vi "Open.vi"(8 "error in (no error)":errorcluster) -> (0 "error out":errorcluster, 3 "return type":i16)   [LabVIEW 2023]
uses:
  ps2000.dll
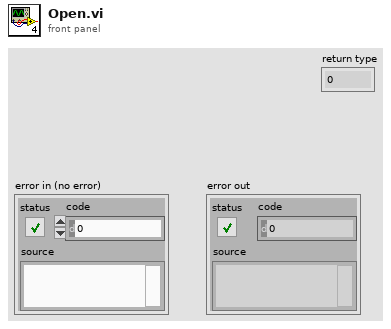
[diagram p1: front panel]
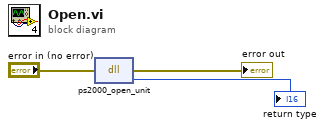
[diagram p0: block diagram]
diagram:
  n1 = dll-call lib="C:/Users/cesar/Desktop/Ps2000 libreria/PS2000.dll" fn="ps2000_open_unit"(error in="error in (no error)") -> (error out=→"error out":errorcluster, "return type"=→"return type":i16)  [unwired: 2 in, 1 out]
